vi "Load Data Preview.V0.54.vi"(4 "Y-Array":dbl[](array[numeric]) format="%.2f", 5 "X-Array":dbl[](array[numeric]) format="%.2f", 7 "File Contents":string, 9 "File Path":path) -> (0 "Continue?":bool, 2 "WL unit copy":i32(ring)=1 items=["Wavelength", "nm", "eV", "meV", "cm-1"])   [LabVIEW 2019]
panel:
  out "?":T1(graph)
  in  "Cancel":bool
  in  "Continue?":bool
  in  "WL unit":i32(ring)=1 items=["Wavelength", "nm", "eV", "meV", "cm-1"]
  # "Please double check the file,\nif it contains valid data, \nselect the wavelength unit \nUSED IN THE FILE:"
  # "Hit \"OK\" to load the data\nor \"Cancel\" to abort."
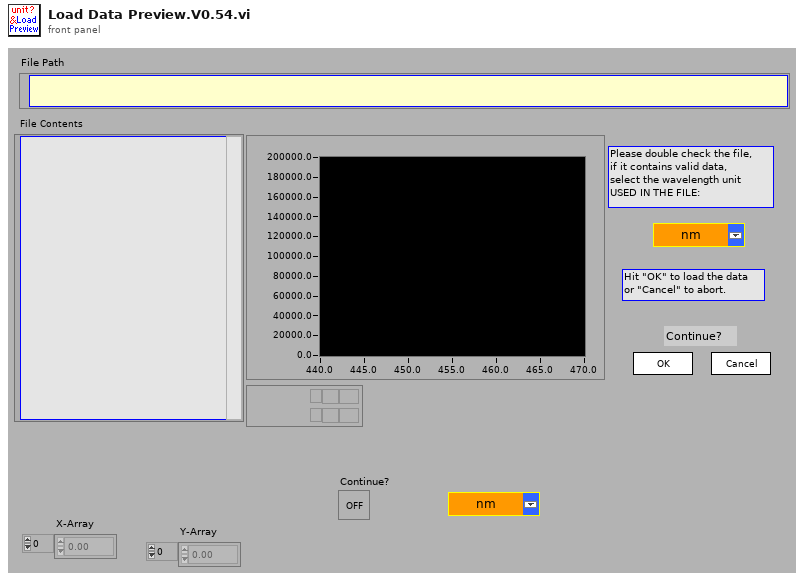
[diagram p1: front panel]
types:
  T1 = cluster{"Ramp Pattern":dbl[], "Sinc Pattern":dbl[]}
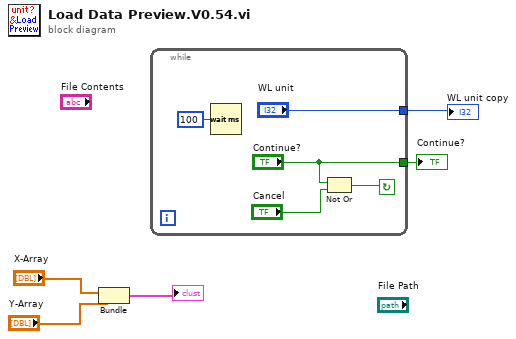
[diagram p0: block diagram]
diagram:
  n1 = Bundle("X-Array"="X-Array", "Y-Array"="Y-Array") -> (→"?":cluster{"X-Array":dbl[], "Y-Array":dbl[]})  [unwired: 1 in]
  n2 = while {
    tunnel: ["Continue?"] -> w4
    tunnel: ["WL unit"] -> w5
    stop <- w10 continue-if-true
    n3 = Wait (ms)(milliseconds to wait=u32 100) -> ()  [unwired: 1 out]
    n4 = Not Or(1:"Cancel", 2:"Continue?") -> (0:w10:bool)
  }
  "WL unit copy" <- w5
  "Continue?" <- w4
